vi "Test Next Name Correct for Case in Suite.vi"(8 "error in (no error)":errorcluster, 11 "Test Case In":refnum<class "Runnable Next Test.lvclass">) -> (0 "error out":errorcluster, 3 "Test Case Out":refnum<class "Runnable Next Test.lvclass">)   [LabVIEW 2020, in "Runnable Next Test.lvclass"]
uses:
  Runnable Next Test/Runnable Next Test.lvclass
  C:/Program Files (x86)/National Instruments/LabVIEW 2020/vi.lib/Astemes/LUnit/Test Case.lvclass
  Test Doubles/Test Case Test Double/Methods.ctl
  <vilib>/Astemes/LUnit/Test Case.lvclass/Test Case.ctl
  e8c5eeff-a694-4c0d-b261-74e2e6f5327d.vi
  <vilib>/Astemes/LUnit/Append Pass Result.vi
  <vilib>/Astemes/LUnit/Append Fail Result.vi
  <vilib>/Astemes/LUnit/Compare Variants.vi
  <vilib>/Astemes/LUnit/Describe Comparison.vi
  <vilib>/Astemes/LUnit/Variant to string.vi
  source/API/LUnit Test Case/LUnit Test Case.lvclass
  C:/git/astemes-lunit/source/Core/Runnable/Runnable.lvclass
  <vilib>/Utility/Data Type/Get Type Information.vi
  <vilib>/Utility/LVClass/Get LV Class Name.vi
  source/API/LUnit Test Suite/LUnit Test Suite.lvclass
  Test Doubles/Test Case Test Double/Test Case Test Double.lvclass
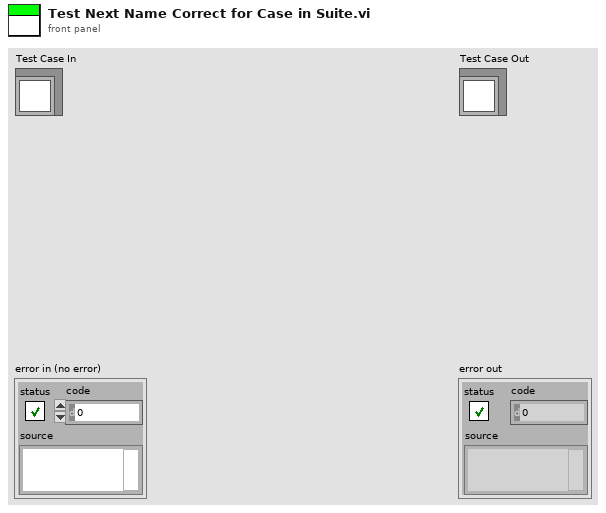
[diagram p1: front panel]
types:
  T1 = typedef "Test Case Test Double.lvclass/Methods.ctl" = enum16{"Test Failing Test.vi", "Test Passing Test.vi", "Test Error Test.vi", "Test Skip Test.vi", "Test Passing Pass If Test.vi", "Test Failing Pass If Test.vi", "Test Failing Fail If Test.vi", "Test Passing Fail If Test.vi", "Test Passing Pass If Error Test.vi", "Test Failing Pass If Error Test.vi", "Test Passing Fail If Error Test.vi", "Test Failing Fail If Error Test.vi", "Test Passing Pass If Equal Test.vi", "Test Failing Pass If Equal Test.vi", "Test Failing Fail If Equal Test.vi", "Test Passing Fail If Equal Test.vi", "Freezing Test.vi"}
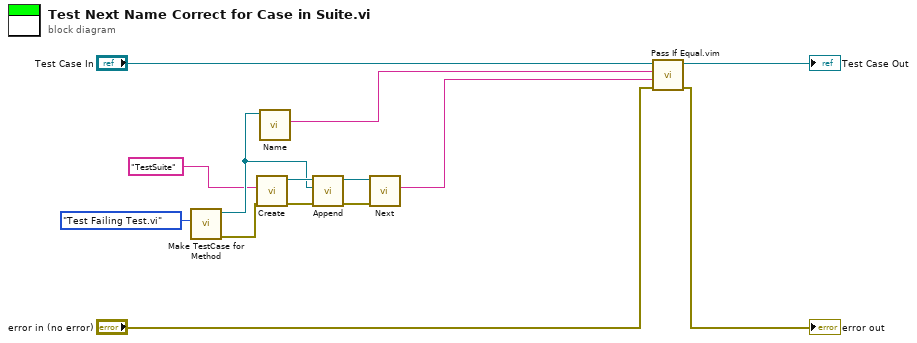
[diagram p0: block diagram]
diagram:
  n1 = call "Make TestCase for Method.vi"("Test Method"=Methods."Test Failing Test.vi") -> ("error out"=w9:errorcluster, "LUnit Test Case V2 out"=w3:refnum<class "LUnit Test Case.lvclass">)  [unwired: 9 in]
  n2 = call "Create.vi"("error in (no error)"=w9, "Suite Name"="TestSuite") -> ("error out"=w6:errorcluster, "LUnit Test Suite Out"=w4:refnum<class "LUnit Test Suite.lvclass">)  [unwired: 8 in]
  n3 = call-dynamic "Name.vi"("LUnit Test Case in"=w3) -> ("Name"=w7:string)  [unwired: 8 in, 2 out]
  n4 = call "Append.vi"("error in (no error)"=w6, "Runnable"=w3, "LUnit Test Suite In"=w4) -> ("error out"=w5:errorcluster, "LUnit Test Suite Out"=w1:refnum<class "LUnit Test Suite.lvclass">)  [unwired: 7 in]
  n5 = call-dynamic "Next.vi"("error in (no error)"=w5, "LUnit Test Suite In"=w1) -> ("Name"=w8:string)  [unwired: 6 in, 3 out]
  n6 = call "Pass If Equal.vim"("error in (no error)"="error in (no error)", "Actual"=w8, "Expected"=w7, "LUnit Test Case In"="Test Case In") -> ("error out"=→"error out":errorcluster, "LUnit Test Case Out"=→"Test Case Out":refnum<class "Runnable Next Test.lvclass">)  [unwired: 6 in]
